vi "Replace zeroes if not stopping 4x motors.vi"(0 "Motor 1 in":dbl, 1 "Stop?":bool, 5 "Motor 2 in":dbl, 7 "Motor 3 in":dbl, 9 "Motor 4 in":dbl, 11 "error in (no error)":errorcluster) -> (4 "Motor 1 out":dbl, 6 "Motor 2 out":dbl, 8 "Motor 3 out":dbl, 10 "Motor 4 out":dbl, 15 "error out":errorcluster)   [LabVIEW 2017]
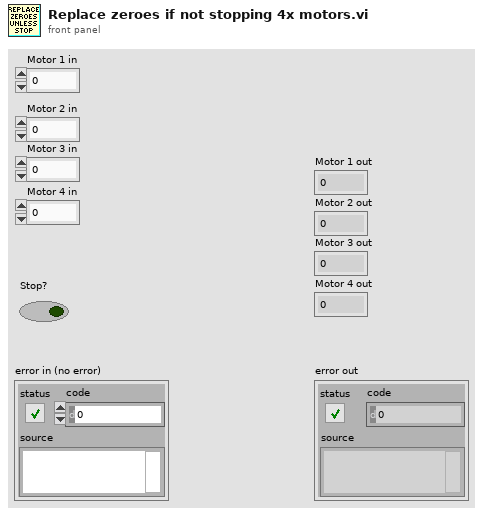
[diagram p1: front panel]
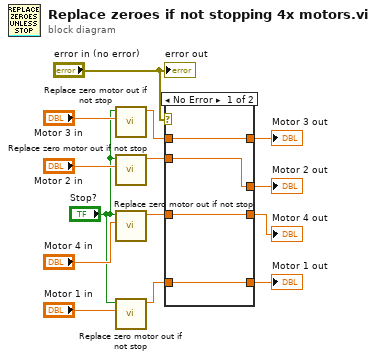
[diagram p0: block diagram]
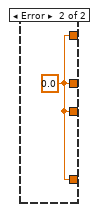
[diagram p2: hidden frame]
diagram:
  n1 = call "Replace zero motor out if not stop.vi"("Input"="Motor 3 in", "Stop?"="Stop?") -> ("Output"=w5:dbl)  [unwired: 9 in]
  n2 = call "Replace zero motor out if not stop.vi"("Input"="Motor 2 in", "Stop?"="Stop?") -> ("Output"=w7:dbl)  [unwired: 9 in]
  n3 = call "Replace zero motor out if not stop.vi"("Input"="Motor 4 in", "Stop?"="Stop?") -> ("Output"=w3:dbl)  [unwired: 9 in]
  n4 = call "Replace zero motor out if not stop.vi"("Input"="Motor 1 in", "Stop?"="Stop?") -> ("Output"=w9:dbl)  [unwired: 9 in]
  n5 = case shown="No Error" "error in (no error)" {
    tunnel: w9 -> [w18 _]
    tunnel: [w18 w19] -> w8
    tunnel: w7 -> [w17 _]
    tunnel: [w17 w19] -> w6
    tunnel: w5 -> [w16 _]
    tunnel: [w16 w19] -> w4
    tunnel: w3 -> [w15 _]
    tunnel: [w15 w19] -> w2
    frame No Error {
    }
    frame Error {
      w19 = 0.0 ("Output")
    }
  }
  "Motor 1 out" <- w8
  "Motor 2 out" <- w6
  "Motor 3 out" <- w4
  "Motor 4 out" <- w2
  "error out" <- "error in (no error)"
